vi "Close POP session.vi"(1 "error in (no error)":errorcluster, 2 "connection ID":refnum<k5>) -> (0 "error out":errorcluster)   [LabVIEW 2012]
doc: "This VI simply closes the TCP/IP connection to the mail server machine."
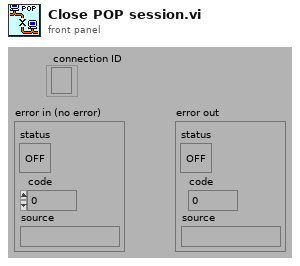
[diagram p1: front panel]
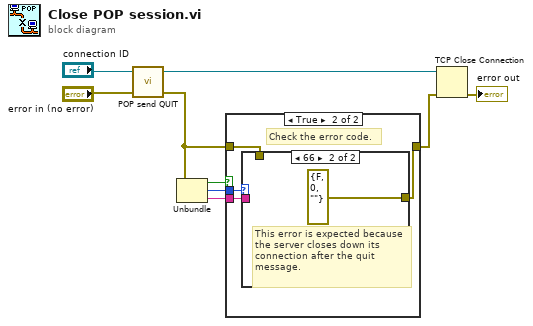
[diagram p0: block diagram]
diagram:
  n1 = call "POP send QUIT.vi"("error in"="error in (no error)", "connection ID in"="connection ID") -> ("error out"=w2:errorcluster, "connection ID out"=w8:refnum<k5>)  [unwired: 1 in, 1 out]
  n2 = Unbundle(w2) -> ("status"=w5:bool, "code"=w4:i32, "source"=w3:string)
  n3 = case shown="True" w5 {
    tunnel: w4 -> [_ w14]
    tunnel: w3 -> [_ w13]
    tunnel: w2 -> [w10 w12]
    tunnel: [w10 w11] -> w1
    frame False {
      # "No error, continue on."
    }
    frame True {
      # "Check the error code."
      n4 = case shown="66" w14 {
        tunnel: w13 -> [_ _]
        tunnel: [w15 errorcluster {"status"=FALSE, "code"=0, "source"=""} ("error out")] -> w11
        tunnel: w12 -> [w15 _]
        frame 0, Default {
          # "Pass any other error number\nalong to be dealt with."
        }
        frame 66 {
          # "This error is expected because\nthe server closes down its\nconnection after the quit\nmessage."
        }
      }
    }
  }
  n5 = TCP Close Connection(connection ID=w8, error in (no error)=w1) -> (error out=→"error out":errorcluster)  [unwired: 1 in, 1 out]
